vi "Destroy.vi"(8 "Error In":errorcluster, 11 "KnownHosts":refnum<class "KnownHosts.lvclass">) -> (0 "Error Out":errorcluster)   [LabVIEW 2017, in "Toolkit.lvlib" / "KnownHosts.lvclass"]
uses:
  KnownHosts.lvclass
  KnownHosts.lvclass/KnownHosts.ctl
  Toolkit.lvlib
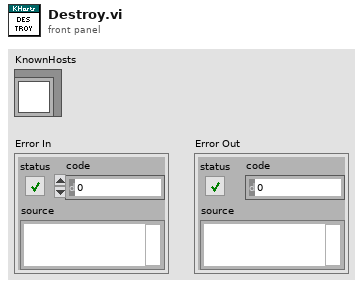
[diagram p1: front panel]
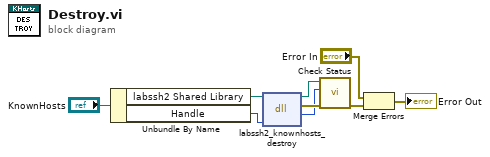
[diagram p0: block diagram]
diagram:
  n1 = Unbundle By Name("KnownHosts") -> ("labssh2 Shared Library"=w6:path, "Handle"=w5:u64)
  n2 = dll-call lib="D:/Users/cfield/Code/Field R&D Services/SSH/LabSSH2/LabVIEW/trunk/src/LabSSH2/Private/labssh2.*" fn="labssh2_knownhosts_destroy"(path in=w6, "handle"=w5) -> (path out=w3:path, error out=w4:errorcluster, "status"=w2:i32)  [unwired: 3 in]
  n3 = call "Check Status.vi"("Error In"=w4, "Status"=w2, "labssh2 Shared Library In"=w3) -> ("Error Out"=w1:errorcluster)  [unwired: 7 in, 1 out]
  n4 = Merge Errors("Error In", w1) -> (→"Error Out":errorcluster)
